vi "[FPGA] eHS Main (9039).vi"() -> ()   [LabVIEW 2017]
uses:
  <vilib>/OPAL-RT/eHS Toolkit/eHS Common/Controls/eHSx64 Gen3 Configuration.ctl
  <vilib>/OPAL-RT/Utilities Toolkit/Mapping/Input Mapping/FPGA/Controls/Input Mapping Configuration FIFO.ctl
  <vilib>/OPAL-RT/Utilities Toolkit/Mapping/Switch Mapping/FPGA/Controls/Switch Mapping Configuration FIFO.ctl
  <vilib>/OPAL-RT/Analog I-O Mapping & Conditioning Toolkit/AOMC/FPGA/Public/Controls/AOMC Configuration FIFO.ctl
  <vilib>/Platform/TimedLoop/XDataNode/timing_clust.ctl
  <vilib>/Platform/TimedLoop/XDataNode/nitl_modes.ctl
  <vilib>/Platform/TimedLoop/XDataNode/wakeup.ctl
  <vilib>/OPAL-RT/Analog I-O Mapping & Conditioning Toolkit/AIC/FPGA/Public/Controls/AIC Configuration FIFO.ctl
  <vilib>/OPAL-RT/FPGA Signal Generation Toolkit/Sinewave Generation/FPGA/Public/Controls/Sinewave Configuration FIFO.ctl
  <vilib>/OPAL-RT/FPGA Signal Generation Toolkit/SPWM Generation/FPGA/Public/Controls/SPWM Configuration FIFO.ctl
  <vilib>/OPAL-RT/FPGA Signal Generation Toolkit/PWM Generation/FPGA/Public/Controls/PWM Configuration FIFO.ctl
  <vilib>/OPAL-RT/Analog I-O Mapping & Conditioning Toolkit/AOMC/FPGA/Public/Controls/Input Sources.ctl
  <vilib>/OPAL-RT/Utilities Toolkit/Mapping/Input Mapping/FPGA/Controls/Sources/Input Sources - Parallelx32.ctl
  <vilib>/OPAL-RT/Utilities Toolkit/Mapping/Switch Mapping/FPGA/Controls/Sources/Switch Sources - Parallelx72.ctl
  <vilib>/rvi/Emulation/niFpgaGetClockAttributes.vi
  <vilib>/rvi/Emulation/niFpgaSctlEmulationGetInTimedLoop.vi
  <vilib>/rvi/Emulation/niFpgaEmulationReportErrorSimple.vi
  <vilib>/OPAL-RT/Utilities Toolkit/Mapping/Input Mapping/FPGA/SubVIs/Initialize/Initialize Input Mapping - Parallelx32.vi
  <vilib>/OPAL-RT/Utilities Toolkit/Mapping/Switch Mapping/FPGA/SubVIs/Initailize/Initialize Switch Mapping - Parallelx72.vi
  <vilib>/rvi/DataTransferAndStorage/Container/Common/niFpgaContainerExecOnDevCompGetState.vi
  <vilib>/rvi/Emulation/niFpgaEmulationIsFPGAContextNoSignature.vi
  <vilib>/rvi/DataTransferAndStorage/Container/Common/niFpgaContainerGetUniqueNameForEmu.vi
  <vilib>/rvi/Memory/Memory_Emulation/niFpgaMemoryEmulationCacheClearOnFirstRun.vi
  <vilib>/rvi/Memory/Memory_Emulation/nirvimemoryEmulationManagerCache_MakeExclusive.vi
  <vilib>/rvi/Memory/Memory_Emulation/niFpgaMemoryEmulationValidateCache.vi
  <vilib>/rvi/Memory/Memory_Emulation/nirvimemoryEmulationManagerCache_InsertValue.vi
  <vilib>/Utility/error.llb/Clear Errors.vi
  <vilib>/rvi/Memory/Memory_Emulation/nirvimemoryEmulationManagerCache_ReleaseExclusive.vi
  <vilib>/rvi/Memory/Memory_Emulation/nirvimemoryEmulationManagerCache_GetValue.vi
  <vilib>/rvi/Memory/Memory_Emulation/nirvimemoryEmulationManagerCache_SetValue.vi
  <vilib>/rvi/Emulation/niFpgaProcessEmulError.vi
  <vilib>/rvi/eio/common/nirviEmuTemplateMethod_errors.vi
  <vilib>/rvi/Emulation/niFpgaCriticalErrorInLSC.vi
  <vilib>/OPAL-RT/FPGA Signal Generation Toolkit/Sinewave Generation/FPGA/Private/Generators/Sinewave Generators (32-CH Parallel).vi
  <vilib>/OPAL-RT/FPGA Signal Generation Toolkit/SPWM Generation/FPGA/Private/Generators/SPWM Generators (12-CH Parallel).vi
  <vilib>/OPAL-RT/FPGA Signal Generation Toolkit/PWM Generation/FPGA/Private/Generators/PWM Generators (16-CH Parallel).vi
  <vilib>/OPAL-RT/Analog I-O Mapping & Conditioning Toolkit/AOMC/FPGA/Private/AO Mapping & Conditioning (FXP(20,5)).vi
  <vilib>/OPAL-RT/Analog I-O Mapping & Conditioning Toolkit/AIC/FPGA/Private/AI Conditioning FXP(20,5).vi
  <vilib>/OPAL-RT/eHS Toolkit/eHS FPGA/SubVIs/eHSx64 Gen3 Solver Core.vi
  <vilib>/OPAL-RT/Utilities Toolkit/Mapping/Switch Mapping/FPGA/SubVIs/Configure/Get Switch Mapping Configuration from Host - Parallelx72.vi
  <vilib>/OPAL-RT/Utilities Toolkit/Mapping/Input Mapping/FPGA/SubVIs/Configure/Get Input Mapping Configuration from Host - Parallelx32.vi
  <vilib>/OPAL-RT/Utilities Toolkit/Mapping/Switch Mapping/FPGA/SubVIs/Map/Map Switches - Parallelx72.vi
  <vilib>/OPAL-RT/Utilities Toolkit/Mapping/Input Mapping/FPGA/SubVIs/Map/Map Inputs - Parallelx32.vi
  <vilib>/rvi/interface/RandomDataEmulation/niFpgaRandomDataHandleErrors.vi
  <vilib>/Platform/TimedLoop/XDataNode/XDataNode.xnode
  <vilib>/rvi/DataTransferAndStorage/Container/XNode/niFpgaContainer.xnode
  <vilib>/rvi/DataTransferAndStorage/Register/Emulation/niFpgaRegisterEmulationRefIn.vi
  <vilib>/eio/EIONode/EIONode.xnode
  <vilib>/rvi/interface/RandomDataEmulation/nirviRandomDataFpgaReadWriteTemplate.vi
  <vilib>/Platform/TimedLoop/XDataNode/XDNodeRunTimeDep.lvlib
  <vilib>/OPAL-RT/Utilities Toolkit/Mapping/Input Mapping/FPGA/Input Mapping - FPGA.lvlib
  <vilib>/OPAL-RT/Utilities Toolkit/Mapping/Switch Mapping/FPGA/Switch Mapping - FPGA.lvlib
  <vilib>/OPAL-RT/Analog I-O Mapping & Conditioning Toolkit/AOMC/FPGA/AO Mapping & Conditioning - FPGA.lvlib
  <vilib>/OPAL-RT/Analog I-O Mapping & Conditioning Toolkit/AIC/FPGA/AI Conditioning - FPGA.lvlib
  <vilib>/OPAL-RT/eHS Toolkit/eHS FPGA/eHS - FPGA.lvlib
  <vilib>/OPAL-RT/Utilities Toolkit/Utilities/Type Casting/FPGA/Type Casting - FPGA.lvlib
  <vilib>/OPAL-RT/FPGA Signal Generation Toolkit/Sinewave Generation/FPGA/Sinewave Generation - FPGA.lvlib
  <vilib>/OPAL-RT/FPGA Signal Generation Toolkit/SPWM Generation/FPGA/SPWM Generation - FPGA.lvlib
  <vilib>/OPAL-RT/FPGA Signal Generation Toolkit/PWM Generation/FPGA/PWM Generation - FPGA.lvlib
  <vilib>/OPAL-RT/eHS Toolkit/eHS Common/eHS - Common.lvlib
panel:
  in  "View SPWM":bool
  in  "Mod Index":fxp<+/-,32,2>
  in  "Carrier Frequency":fxp<+/-,32,1>=0.00039999978616833687
  in  "Reset Sinewaves?":bool
  in  "Auto-Synchronize Sinewaves?":bool
  in  "Auto-Synchronize SPWM?":bool
  in  "Reset SPWMs?":bool
  in  "Reset PWMs?":bool
  out "Conditioned AI Data_Debug":sgl[](array[numeric])
  out "Mapped & Conditioned Data_Debug":fxp<+/-,20,5>[](array[numeric])
  in  "eHS Switches (CPU)":bool[](array[boolean])=[FALSE, FALSE, FALSE, FALSE, FALSE, FALSE, FALSE, FALSE, FALSE, FALSE, FALSE, FALSE, FALSE, FALSE, FALSE, FALSE, FALSE, FALSE, FALSE, FALSE, FALSE, FALSE, FALSE, FALSE, FALSE, FALSE, FALSE, FALSE, FALSE, FALSE, FALSE, FALSE, FALSE, FALSE, FALSE, FALSE, FALSE, FALSE, FALSE, FALSE, FALSE, FALSE, FALSE, FALSE, FALSE, FALSE, FALSE, FALSE, FALSE, FALSE, FALSE, FALSE, FALSE, FALSE, FALSE, FALSE, FALSE, FALSE, FALSE, FALSE, FALSE, FALSE, FALSE, FALSE, FALSE, FALSE, FALSE, FALSE, FALSE, FALSE, FALSE, FALSE]
  in  "eHS Input (CPU)":u32[](array[numeric])=[0, 0, 0, 0, 0, 0, 0, 0, 0, 0, 0, 0, 0, 0, 0, 0, 0, 0, 0, 0, 0, 0, 0, 0, 0, 0, 0, 0, 0, 0, 0, 0]
  in  "eHSx64 Gen3 Configuration":T1
  out "Finished":bool
  in  "stop":bool
  out "Module Underflow":bool
  out "Acq Loop Ticks":u32
  out "DMA FIFO Full":bool
  out "Chan Count":bool
  out "First Read":bool
  in  "Number of Channels":i32=4
  in  "Samps per Chan [Finite]":i32=5120
  in  "Acquisition Type":enum16{"Finite Samples", "Continuous Samples"}(ring)
  out "oclk div":u32
  out "oclk freq":u32
  in  "data rate (S/s)":u32
  out "oclk mult":u32
  out "FPGA Error":errorcluster
  in  "Chan Scale Array":sgl[](array[numeric])=[0.0, 0.0, 0.0, 0.0, 0.0, 0.0, 0.0, 0.0, 0.0, 0.0, 0.0, 0.0, 0.0, 0.0, 0.0, 0.0, 0.0, 0.0, 0.0, 0.0, 0.0, 0.0, 0.0, 0.0, 0.0, 0.0, 0.0, 0.0, 0.0, 0.0, 0.0, 0.0, 0.0, 0.0, 0.0, 0.0, 0.0, 0.0, 0.0, 0.0]
  # "Signal Generation Paramters"
  # "eHS Parameters"
  # "RIO Waveform Parameters"
  # "Debug"
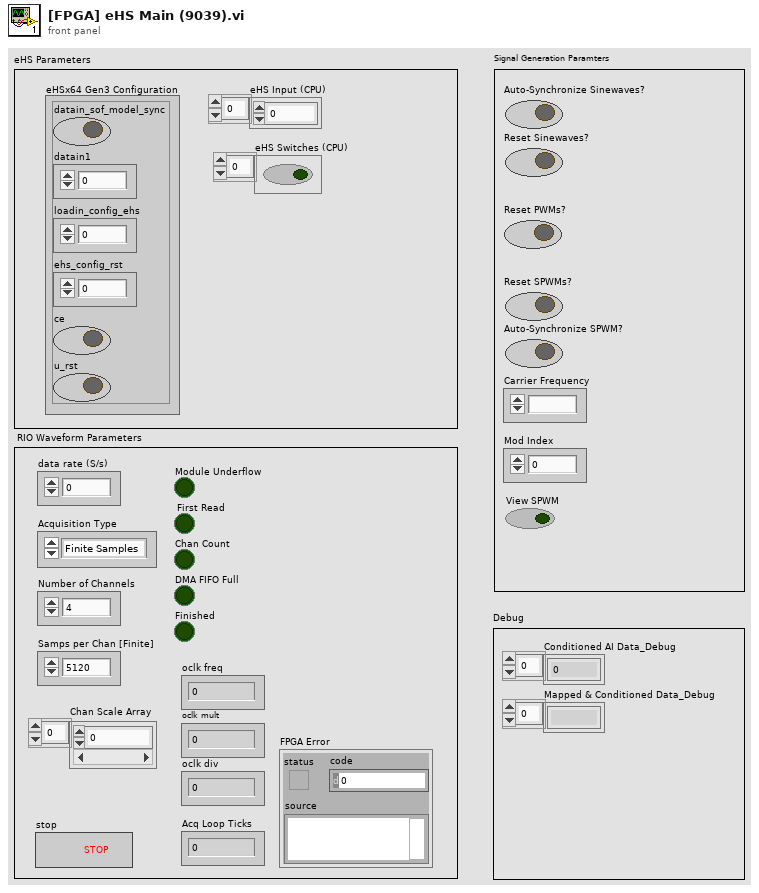
[diagram p1: front panel]
types:
  T1 = typedef "OPAL-RT eHS.lvlib/eHS - Common.lvlib/eHSx64 Gen3 Configuration.ctl" = cluster{"datain_sof_model_sync":bool, "datain1":fxp<+,33,33>, "loadin_config_ehs":fxp<+,33,33>, "ehs_config_rst":fxp<+,33,33>, "ce":bool, "u_rst":bool}
  T2 = typedef "PWM Generation - FPGA.lvlib/PWM Configuration FIFO.ctl" = refnum<k21>
  T3 = typedef "SPWM Generation - FPGA.lvlib/SPWM Configuration FIFO.ctl" = refnum<k21>
  T4 = typedef "Sinewave Generation - FPGA.lvlib/Sinewave Configuration FIFO.ctl" = refnum<k21>
  T5 = typedef "AI Conditioning - FPGA.lvlib/AIC Configuration FIFO.ctl" = refnum<k21>
  T6 = typedef "AO Mapping & Conditioning - FPGA.lvlib/AOMC Configuration FIFO.ctl" = refnum<k21>
  T7 = typedef "Switch Mapping - FPGA.lvlib/Switch Mapping Configuration FIFO.ctl" = refnum<k21>
  T8 = typedef "Input Mapping - FPGA.lvlib/Input Mapping Configuration FIFO.ctl" = refnum<k21>
  T9 = typedef "[FPGA] Local FPGA Memory.ctl" = cluster{"Analog Inputs":refnum<k21>, "Conditioned AI":refnum<k21>, "Analog Outputs (FXP(20,5))":refnum<k21>, "Analog Outputs (U16)":refnum<k21>, "Digital Inputs":refnum<k21>, "Digital Outputs":refnum<k21>, "eHS Outputs - Lane 1":refnum<k21>, "eHS Outputs - Lane 2":refnum<k21>, "eHS Outputs - Lane 3":refnum<k21>, "SWG Signals":refnum<k21>, "PWM Signals":refnum<k21>, "SPWM Signals":refnum<k21>}
  T10 = typedef "XDNodeRunTimeDep.lvlib/timing_clust.ctl" = cluster{"Expected End [f-1]":u64, "Actual End [f-1]":u64, "Finished Late? [f-1]":bool, "Expected End [i-1]":u64, "Actual End [i-1]":u64, "Finished Late? [i-1]":bool, "Expected Start [i]":u64, "Actual Start [i]":u64, "Expected Start [f]":u64, "Actual Start [f]":u64, "Source Name":string, "Structure Name":string, "Period":i64, "Deadline":i64, "Offset":i64, "Start":i64, "Priority":i32, "Timeout":i32, "Mode":T11, "Wakeup Reason":T12, "Error":errorcluster, "Source Type":string, "Secondary Source Type":string, "Global End Time":u64, "Global Start Time":u64, "Frame Duration":u64, "Iteration Duration":u64, "Assigned CPU":i32, "I/O Scan Engine Mode":u32}
  T11 = typedef "XDNodeRunTimeDep.lvlib/nitl_modes.ctl" = enum32{"No Change", "Process missed periods, maintain original phase", "Discard missed periods, maintain original phase", "Process missed periods, ignore original phase", "Discard missed periods, ignore original phase"}
  T12 = typedef "XDNodeRunTimeDep.lvlib/wakeup.ctl" = enum32{"Normal", "Aborted", "Asynchronous wakeup", "Timing source error", "Timed loop error", "Timeout"}
  T13 = typedef "Sinewave Generation - FPGA.lvlib/Sinewave Generator FPGA Resources.ctl" = cluster{"Sinewave Configuration FIFO":T4, "Sinewave Configuration Memory":T14}
  T14 = typedef "Sinewave Generation - FPGA.lvlib/Sinewave Generator Memory.ctl" = cluster{"Sinewave Generator Configuration Memory":cluster{"Sinewave Generator Configuration - Buffer 0":refnum<k21>, "Sinewave Generator Configuration - Buffer 1":refnum<k21>}, "Frequency Engine Rate Memory":T15, "Frequency Engine Values Memory":T16, "Sinewave LUT Memory":T17}
  T15 = typedef "Signal Generation Utilities - FPGA.lvlib/Frequency Engine Rate Memory.ctl" = cluster{"Frequency Engine Rates - Buffer 0":refnum<k21>, "Frequency Engine Rates - Buffer 1":refnum<k21>}
  T16 = typedef "Signal Generation Utilities - FPGA.lvlib/Frequency Engine Values Memory.ctl" = cluster{"Frequency Engine Values - Buffer 0":refnum<k21>, "Frequency Engine Values - Buffer 1":refnum<k21>}
  T17 = typedef "Signal Generation Utilities - FPGA.lvlib/Sinewave LUT Memory.ctl" = cluster{"Sinewave LUT (SGL)":refnum<k21>, "Sinewave LUT (16,1)":refnum<k21>}
  T18 = typedef "SPWM Generation - FPGA.lvlib/SPWM Generator FPGA Resources.ctl" = cluster{"SPWM Configuration FIFO":T3, "SPWM Generator Memory":T19}
  T19 = typedef "SPWM Generation - FPGA.lvlib/SPWM Generator Memory.ctl" = cluster{"SPWM Configuration Parameters Memory":T20, "Frequency Engine Rate Memory":T15, "Frequency Engine Values Memory":T16, "Sinewave LUT Memory":T17}
  T20 = typedef "SPWM Generation - FPGA.lvlib/SPWM Configuration Parameters Memory.ctl" = cluster{"SPWM Generator Configuration - Buffer 0":refnum<k21>, "SPWM Generator Configuration - Buffer 1":refnum<k21>}
  T21 = typedef "PWM Generation - FPGA.lvlib/PWM Generator FPGA Resources.ctl" = cluster{"PWM Generator Memory":T22, "PWM Configuration FIFO":T2}
  T22 = typedef "PWM Generation - FPGA.lvlib/PWM Generator Memory.ctl" = cluster{"PWM Generation Configuration":refnum<k21>, "PWM Generator States":refnum<k21>}
  T23 = typedef "Input Mapping - FPGA.lvlib/Input Mapping FPGA Resources.ctl" = cluster{"Input Mapping Configuration FIFO":T8, "Input Mapping Configuration Memory":T24}
  T24 = typedef "Input Mapping - FPGA.lvlib/Input Mapping Configuration Memory.ctl" = cluster{"Input Mapping Memory - Lane 0":refnum<k21>, "Input Mapping Memory - Lane 1":refnum<k21>, "Input Mapping Memory - Lane 2":refnum<k21>, "Input Mapping Memory - Lane 3":refnum<k21>}
  T25 = typedef "Switch Mapping - FPGA.lvlib/Switch Mapping FPGA Resources.ctl" = cluster{"Switch Mapping Configuration FIFO":T7, "Switch Mapping Configuration Memory":T26}
  T26 = typedef "Switch Mapping - FPGA.lvlib/Switch Mapping Configuration Memory.ctl" = cluster{"Switch Mapping Memory - Lane 0":refnum<k21>, "Switch Mapping Memory - Lane 1":refnum<k21>, "Switch Mapping Memory - Lane 2":refnum<k21>, "Switch Mapping Memory - Lane 3":refnum<k21>, "Switch Mapping Memory - Lane 4":refnum<k21>, "Switch Mapping Memory - Lane 5":refnum<k21>, "Switch Mapping Memory - Lane 6":refnum<k21>, "Switch Mapping Memory - Lane 7":refnum<k21>, "Switch Mapping Memory - Lane 8":refnum<k21>}
  T27 = typedef "AI Conditioning - FPGA.lvlib/AIC FPGA Resources.ctl" = cluster{"AIC Configuration FIFO":T5, "AIC Memory":T28}
  T28 = typedef "AI Conditioning - FPGA.lvlib/AIC Memory.ctl" = cluster{"AIC Configuration Parameters":refnum<k21>}
  T29 = typedef "AO Mapping & Conditioning - FPGA.lvlib/AOMC FPGA Resources.ctl" = cluster{"AOMC Memory":T30, "AOMC Configuration FIFO":T6}
  T30 = typedef "AO Mapping & Conditioning - FPGA.lvlib/AOMC Memory.ctl" = cluster{"AOMC Configuration Parameters":refnum<k21>}
  T31 = typedef "Sinewave Generation - FPGA.lvlib/Sinewave Generator Parameters.ctl" = cluster{"Number of Sinewaves to Generate":u8, "Read Buffer Index":u8, "Reset Sinewaves?":bool}
  T32 = typedef "SPWM Generation - FPGA.lvlib/SPWM FPGA Generator Parameters.ctl" = cluster{"Carrier Frequency":fxp<+/-,32,1>, "Mod Index ":fxp<+/-,32,2>, "Number of SPWMs to Generate":u8, "Reset SPWMs?":bool, "Read Buffer Index":u8}
  T33 = typedef "PWM Generation - FPGA.lvlib/PWM Generator Parameters.ctl" = cluster{"Number of PWMs to Generate":u8, "Reset PWMs?":bool}
  T34 = typedef "Switch Mapping - FPGA.lvlib/Switch Sources - Parallelx72.ctl" = cluster{"Group A":bool[], "Group B":bool[], "Group C":bool[], "Group D":bool[], "Group E":bool[]}
  T35 = typedef "Input Mapping - FPGA.lvlib/Input Sources - Parallelx32.ctl" = cluster{"Group A":u32[], "Group B":u32[], "Group C":u32[], "Group D":u32[]}
  T36 = typedef "AO Mapping & Conditioning - FPGA.lvlib/Input Sources.ctl" = cluster{"Group A":sgl[], "Group B":sgl[]}
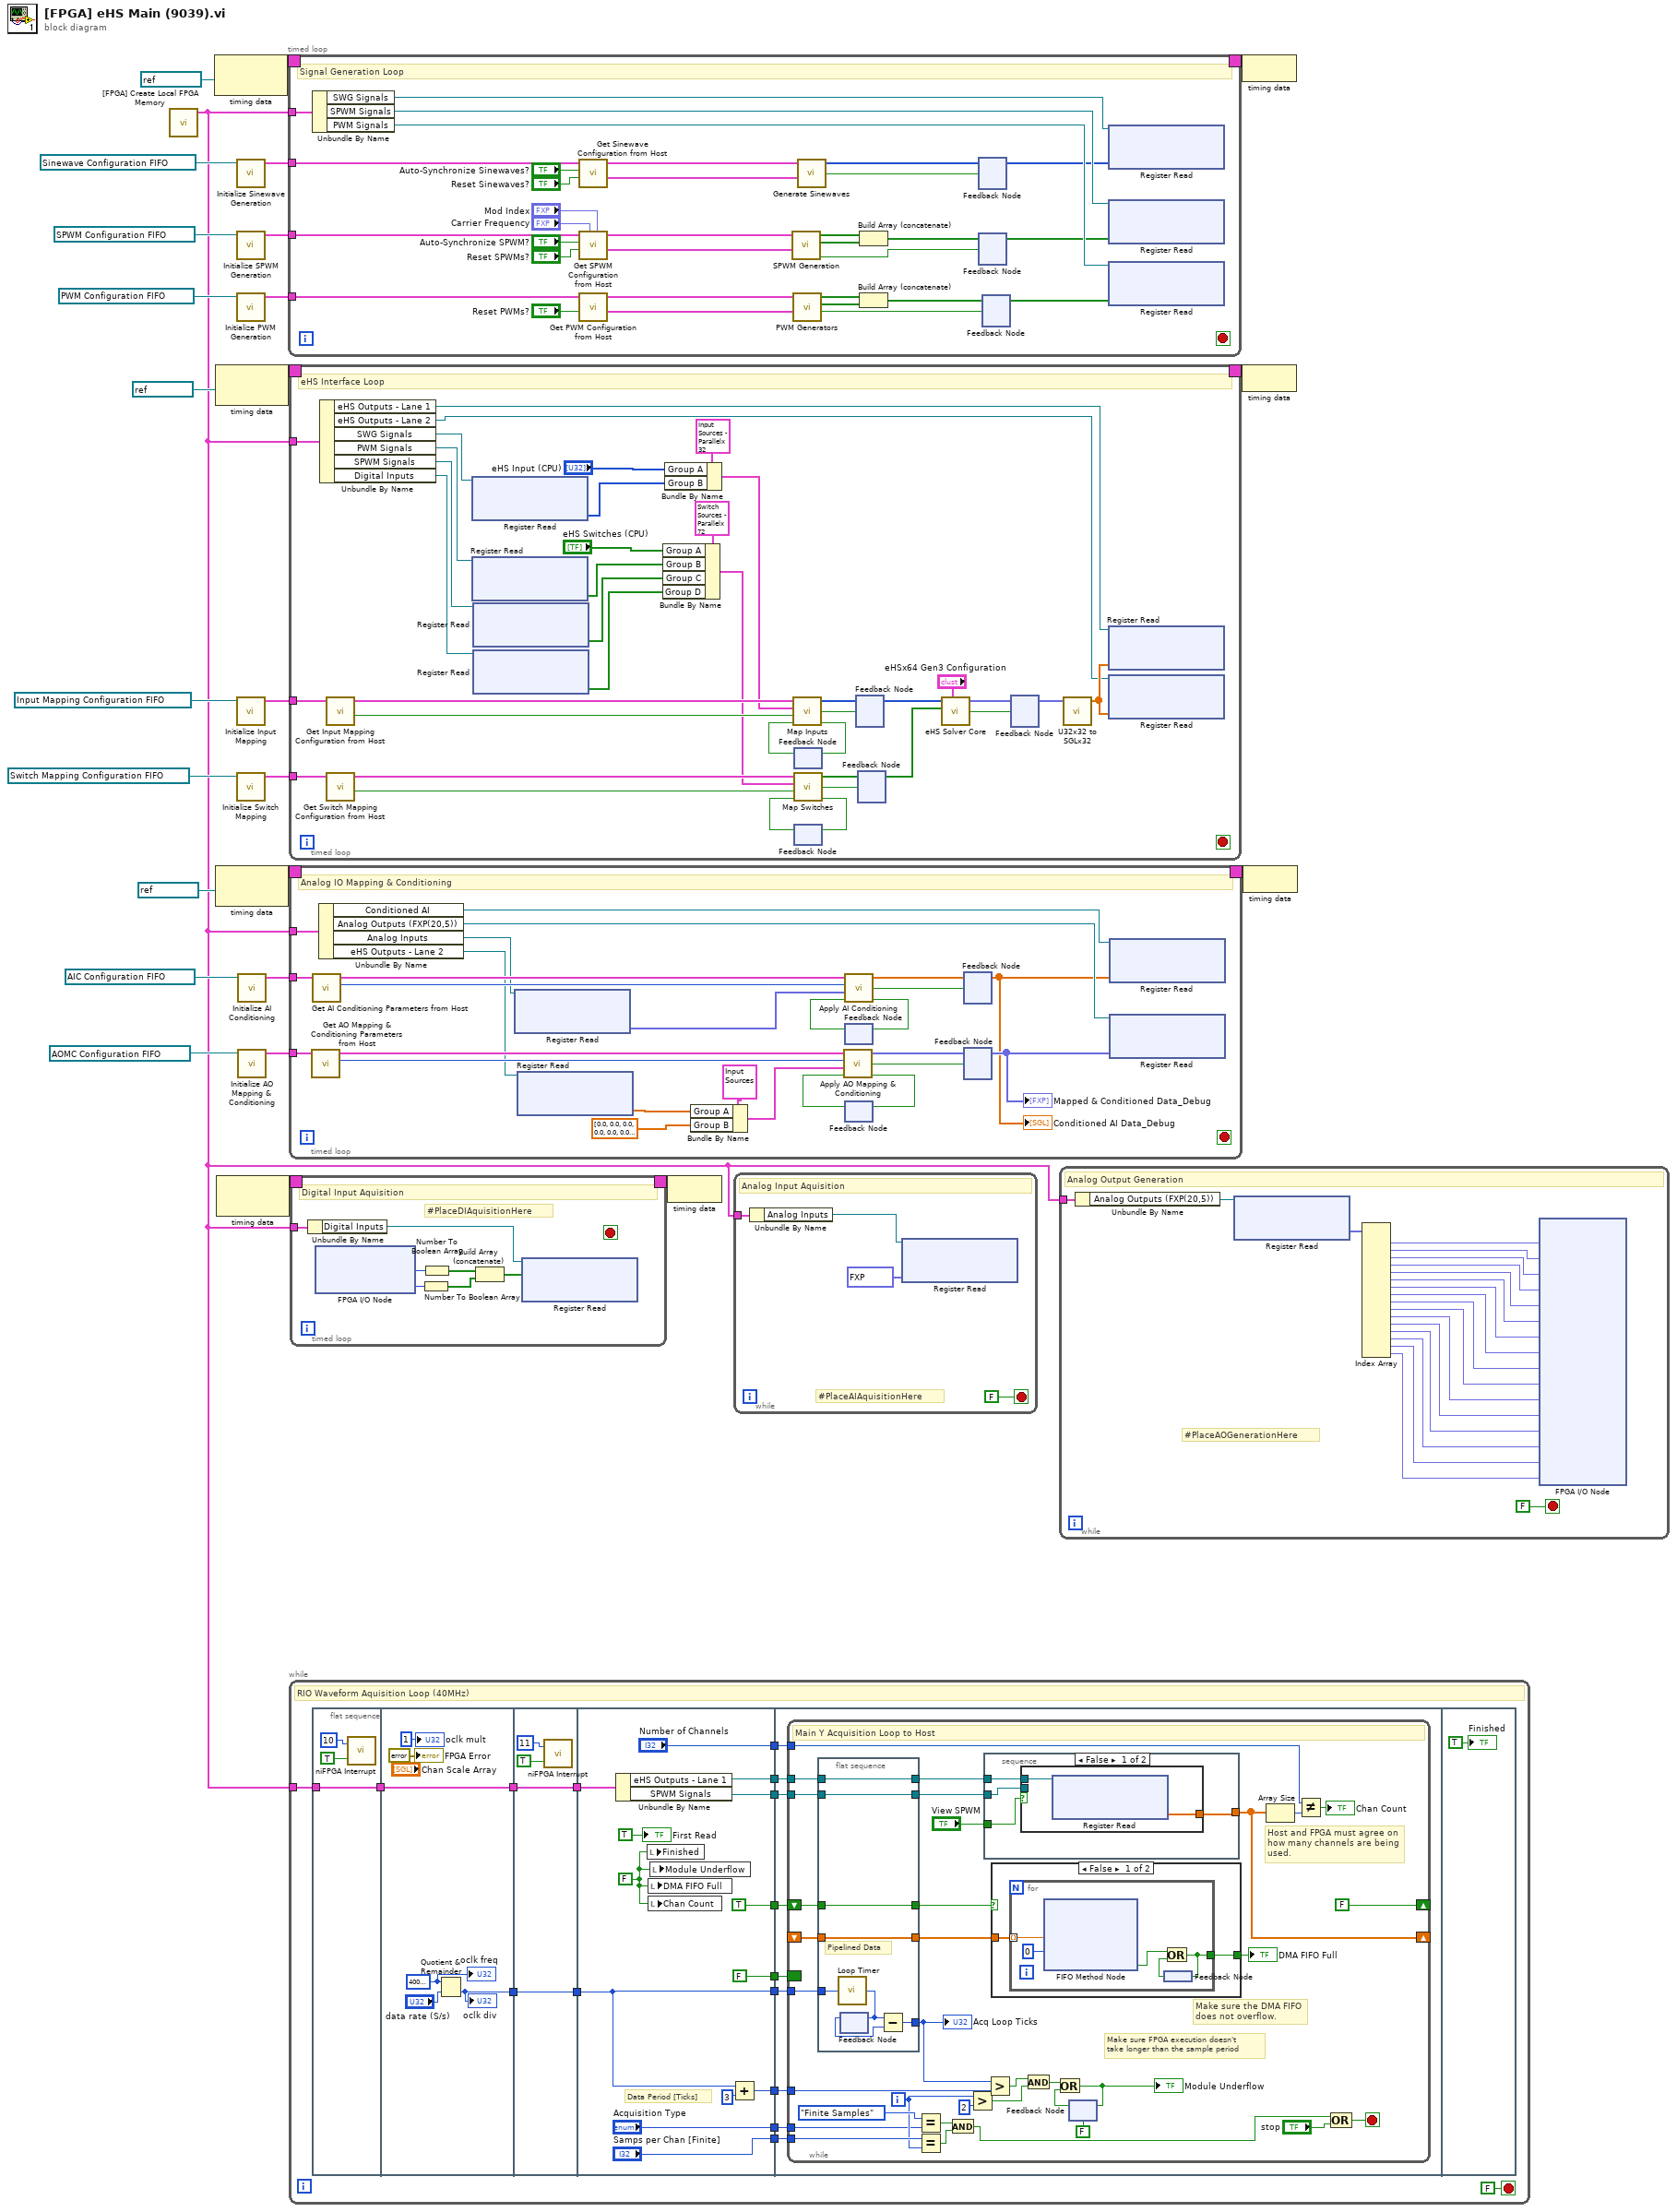
[diagram p0: block diagram]
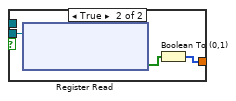
[diagram p2: hidden frame]
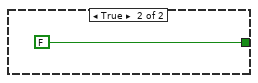
[diagram p3: hidden frame]
diagram:
  n1 = call "[FPGA] Create Local FPGA Memory.vi"() -> ("FPGA Memory"=w1:T9)  [unwired: 11 in]
  n2 = node-c288(refnum<k21> "100MHz" ("Source Name")) -> (w12:T10)
  n3 = node-c288(refnum<k21> "200MHz" ("Source Name")) -> (w26:T10)
  n4 = node-c288(refnum<k21> "200MHz" ("Source Name")) -> (w20:T10)
  n5 = node-c288() -> (w3:T10)  [unwired: 1 in]
  n6 = call <vilib>:"Initialize Sinewave Generation.vi"("Sinewave Configuration FIFO"=T4 "Sinewave Configuration FIFO") -> ("Sinewave Generator FPGA Resources"=w4:T13)  [unwired: 10 in]
  n7 = call <vilib>:"Initialize SPWM Generation.vi"("SPWM Configuration FIFO"=T3 "SPWM Configuration FIFO") -> ("SPWM Generator FPGA Resources"=w5:T18)  [unwired: 10 in]
  n8 = call <vilib>:"Initialize PWM Generation.vi"("PWM Configuration FIFO"=T2 "PWM Configuration FIFO") -> ("PWM Generator FPGA Resources"=w6:T21)  [unwired: 10 in]
  n9 = call-poly <vilib>:"Initialize Input Mapping.vi"("Input Mapping Configuration FIFO"=T8 "Input Mapping Configuration FIFO") -> ("Input Mapping FPGA Resources"=w14:T23)  [unwired: 10 in]
  n10 = call-poly <vilib>:"Initialize Switch Mapping.vi"("Switch Mapping Configuration FIFO"=T7 "Switch Mapping Configuration FIFO") -> ("Switch Mapping FPGA Resources"=w13:T25)  [unwired: 10 in]
  n11 = call <vilib>:"Initialize AI Conditioning.vi"("AIC Configuration FIFO"=T5 "AIC Configuration FIFO") -> ("AIC FPGA Resources"=w16:T27)  [unwired: 10 in]
  n12 = call <vilib>:"Initialize AO Mapping & Conditioning.vi"("AOMC Configuration FIFO"=T6 "AOMC Configuration FIFO") -> ("AOMC FPGA Resources"=w15:T29)  [unwired: 10 in]
  n13 = timed-loop {
    timing: w12 -> [_]
    timing-out: [_] -> w11
    tunnel: w1 -> [w59]
    tunnel: w6 -> [w58]
    tunnel: w5 -> [w57]
    tunnel: w4 -> [w56]
    stop <- _ stop-if-true
    # "Signal Generation Loop"
    n14 = Unbundle By Name(w59) -> ("SWG Signals"=w42:refnum<k21>, "SPWM Signals"=w41:refnum<k21>, "PWM Signals"=w40:refnum<k21>)
    n15 = call <vilib>:"Get Sinewave Configuration from Host.vi"("Reset Sinewaves?"="Reset Sinewaves?", "Auto-Synchronize Sinewaves?"="Auto-Synchronize Sinewaves?", "Sinewave Generator FPGA Resources"=w56) -> ("Sinewave Generator Parameters"=w49:T31, "Sinewave Configuration Memory"=w50:T14)  [unwired: 7 in]
    n16 = call <vilib>:"Get SPWM Configuration from Host.vi"("Mod Index"="Mod Index", "Carrier Frequency"="Carrier Frequency", "Reset SPWMs?"="Reset SPWMs?", "Auto-Synchronize SPWM?"="Auto-Synchronize SPWM?", "SPWM Generator FPGA Resources"=w57) -> ("SPWM Generator Parameters"=w47:T32, "SPWM Generator Memory"=w48:T19)  [unwired: 5 in]
    n17 = call <vilib>:"Get PWM Configuration from Host.vi"("Reset PWMs?"="Reset PWMs?", "PWM Generator FPGA Resources"=w58) -> ("PWM Generator Parameters"=w45:T33, "PWM Generator Memory"=w46:T22)  [unwired: 8 in]
    n18 = call-poly <vilib>:"SPWM Generation.vi"("SPWM Generator Parameters"=w47, "SPWM Generator Memory"=w48) -> ("Output Valid"=w30:bool, "!SPWM States"=w35:bool[], "SPWM States"=w36:bool[])  [unwired: 7 in]
    n19 = call-poly <vilib>:"PWM Generators.vi"("PWM Generator Parameters"=w45, "PWM Generator Memory"=w46) -> ("Output Valid?"=w28:bool, "!PWM States"=w31:bool[], "PWM States"=w32:bool[])  [unwired: 7 in]
    n20 = call-poly <vilib>:"Generate Sinewaves.vi"("Sinewave Generator Parameters"=w49, "Sinewave Generator Memory"=w50) -> ("Output Valid?"=w38:bool, "Sinewave (SGL-as-U32)"=w39:u32[])  [unwired: 8 in]
    n21 = Build Array (concatenate)(w36, w35) -> (w34:bool[])
    n22 = Build Array (concatenate)(w32, w31) -> (w29:bool[])
    n23 = feedback-in #1(w39, w38) -> ()
    n24 = feedback #1() -> (w37:u32[])  [unwired: 1 in]
    n25 = feedback #2() -> (w33:bool[])  [unwired: 1 in]
    n26 = feedback-in #2(w34, w30) -> ()
    n27 = feedback #3() -> (w27:bool[])  [unwired: 1 in]
    n28 = feedback-in #3(w29, w28) -> ()
    n29 = xnode ("Register Read")("Data"=w37, "Register In"=w42) -> ()  [unwired: 1 out]
    n30 = xnode ("Register Read")("Data"=w33, "Register In"=w41) -> ()  [unwired: 1 out]
    n31 = xnode ("Register Read")("Data"=w27, "Register In"=w40) -> ()  [unwired: 1 out]
  }
  n32 = timed-loop {
    timing: w26 -> [_]
    timing-out: [_] -> w25
    tunnel: w1 -> [w78]
    tunnel: w14 -> [w98]
    tunnel: w13 -> [w96]
    stop <- _ stop-if-true
    # "eHS Interface Loop"
    n33 = Unbundle By Name(w78) -> ("eHS Outputs - Lane 1"=w73:refnum<k21>, "eHS Outputs - Lane 2"=w70:refnum<k21>, "SWG Signals"=w69:refnum<k21>, "PWM Signals"=w68:refnum<k21>, "SPWM Signals"=w67:refnum<k21>, "Digital Inputs"=w63:refnum<k21>)
    n34 = call-poly <vilib>:"Get Input Mapping Configuration from Host.vi"("Input Mapping FPGA Resources"=w98) -> ("Settings Updated?"=w89:bool, "Input Mapping Configuration Memory"=w97:T24)  [unwired: 9 in]
    n35 = call-poly <vilib>:"Get Switch Mapping Configuration from Host.vi"("Switch Mapping FPGA Resources"=w96) -> ("Settings Updated?"=w90:bool, "Switch Mapping Configuration Memory"=w91:T26)  [unwired: 9 in]
    n36 = xnode ("Register Read")("Register In"=w69) -> ("Data"=w66:u32[])  [unwired: 1 out]
    n37 = xnode ("Register Read")("Register In"=w68) -> ("Data"=w65:bool[])  [unwired: 1 out]
    n38 = xnode ("Register Read")("Register In"=w67) -> ("Data"=w64:bool[])  [unwired: 1 out]
    n39 = xnode ("Register Read")("Register In"=w63) -> ("Data"=w62:bool[])  [unwired: 1 out]
    n40 = Bundle By Name(cluster=T34 {"Group A"=[FALSE, FALSE, FALSE, FALSE, FALSE, FALSE, FALSE, FALSE, FALSE, FALSE, FALSE, FALSE, FALSE, FALSE, FALSE, FALSE, FALSE, FALSE, FALSE, FALSE, FALSE, FALSE, FALSE, FALSE, FALSE, FALSE, FALSE, FALSE, FALSE, FALSE, FALSE, FALSE, FALSE, FALSE, FALSE, FALSE, FALSE, FALSE, FALSE, FALSE, FALSE, FALSE, FALSE, FALSE, FALSE, FALSE, FALSE, FALSE, FALSE, FALSE, FALSE, FALSE, FALSE, FALSE, FALSE, FALSE, FALSE, FALSE, FALSE, FALSE, FALSE, FALSE, FALSE, FALSE, FALSE, FALSE, FALSE, FALSE, FALSE, FALSE, FALSE, FALSE], "Group B"=[FALSE, FALSE, FALSE, FALSE, FALSE, FALSE, FALSE, FALSE, FALSE, FALSE, FALSE, FALSE, FALSE, FALSE, FALSE, FALSE, FALSE, FALSE, FALSE, FALSE, FALSE, FALSE, FALSE, FALSE, FALSE, FALSE, FALSE, FALSE, FALSE, FALSE, FALSE, FALSE, FALSE, FALSE, FALSE, FALSE, FALSE, FALSE, FALSE, FALSE, FALSE, FALSE, FALSE, FALSE, FALSE, FALSE, FALSE, FALSE, FALSE, FALSE, FALSE, FALSE, FALSE, FALSE, FALSE, FALSE, FALSE, FALSE, FALSE, FALSE, FALSE, FALSE, FALSE, FALSE, FALSE, FALSE, FALSE, FALSE, FALSE, FALSE, FALSE, FALSE], "Group C"=[FALSE, FALSE, FALSE, FALSE, FALSE, FALSE, FALSE, FALSE, FALSE, FALSE, FALSE, FALSE, FALSE, FALSE, FALSE, FALSE, FALSE, FALSE, FALSE, FALSE, FALSE, FALSE, FALSE, FALSE, FALSE, FALSE, FALSE, FALSE, FALSE, FALSE, FALSE, FALSE, FALSE, FALSE, FALSE, FALSE, FALSE, FALSE, FALSE, FALSE, FALSE, FALSE, FALSE, FALSE, FALSE, FALSE, FALSE, FALSE, FALSE, FALSE, FALSE, FALSE, FALSE, FALSE, FALSE, FALSE, FALSE, FALSE, FALSE, FALSE, FALSE, FALSE, FALSE, FALSE, FALSE, FALSE, FALSE, FALSE, FALSE, FALSE, FALSE, FALSE], "Group D"=[FALSE, FALSE, FALSE, FALSE, FALSE, FALSE, FALSE, FALSE, FALSE, FALSE, FALSE, FALSE, FALSE, FALSE, FALSE, FALSE, FALSE, FALSE, FALSE, FALSE, FALSE, FALSE, FALSE, FALSE, FALSE, FALSE, FALSE, FALSE, FALSE, FALSE, FALSE, FALSE, FALSE, FALSE, FALSE, FALSE, FALSE, FALSE, FALSE, FALSE, FALSE, FALSE, FALSE, FALSE, FALSE, FALSE, FALSE, FALSE, FALSE, FALSE, FALSE, FALSE, FALSE, FALSE, FALSE, FALSE, FALSE, FALSE, FALSE, FALSE, FALSE, FALSE, FALSE, FALSE, FALSE, FALSE, FALSE, FALSE, FALSE, FALSE, FALSE, FALSE], "Group E"=[FALSE, FALSE, FALSE, FALSE, FALSE, FALSE, FALSE, FALSE, FALSE, FALSE, FALSE, FALSE, FALSE, FALSE, FALSE, FALSE, FALSE, FALSE, FALSE, FALSE, FALSE, FALSE, FALSE, FALSE, FALSE, FALSE, FALSE, FALSE, FALSE, FALSE, FALSE, FALSE, FALSE, FALSE, FALSE, FALSE, FALSE, FALSE, FALSE, FALSE, FALSE, FALSE, FALSE, FALSE, FALSE, FALSE, FALSE, FALSE, FALSE, FALSE, FALSE, FALSE, FALSE, FALSE, FALSE, FALSE, FALSE, FALSE, FALSE, FALSE, FALSE, FALSE, FALSE, FALSE, FALSE, FALSE, FALSE, FALSE, FALSE, FALSE, FALSE, FALSE]} ("Switch Sources"), "Group A"="eHS Switches (CPU)", "Group B"=w65, "Group C"=w64, "Group D"=w62) -> (w86:T34)
    n41 = Bundle By Name(cluster=T35 {"Group A"=[0, 0, 0, 0, 0, 0, 0, 0, 0, 0, 0, 0, 0, 0, 0, 0, 0, 0, 0, 0, 0, 0, 0, 0, 0, 0, 0, 0, 0, 0, 0, 0], "Group B"=[0, 0, 0, 0, 0, 0, 0, 0, 0, 0, 0, 0, 0, 0, 0, 0, 0, 0, 0, 0, 0, 0, 0, 0, 0, 0, 0, 0, 0, 0, 0, 0], "Group C"=[0, 0, 0, 0, 0, 0, 0, 0, 0, 0, 0, 0, 0, 0, 0, 0, 0, 0, 0, 0, 0, 0, 0, 0, 0, 0, 0, 0, 0, 0, 0, 0], "Group D"=[0, 0, 0, 0, 0, 0, 0, 0, 0, 0, 0, 0, 0, 0, 0, 0, 0, 0, 0, 0, 0, 0, 0, 0, 0, 0, 0, 0, 0, 0, 0, 0]} ("Input Sources"), "Group A"="eHS Input (CPU)", "Group B"=w66) -> (w85:T35)
    n42 = feedback #4() -> (w94:bool)  [unwired: 1 in]
    n43 = call-poly <vilib>:"Map Inputs.vi"("Input Valid?"=w94, "Settings Updated?"=w89, "Input Sources"=w85, "Input Mapping Configuration Memory"=w97) -> ("Ready for Input?"=w95:bool, "Output Valid?"=w84:bool, "Mapped Inputs"=w83:u32[])  [unwired: 5 in]
    n44 = feedback-in #4(w95) -> ()
    n45 = feedback #5() -> (w92:bool)  [unwired: 1 in]
    n46 = call-poly <vilib>:"Map Switches.vi"("Input Valid?"=w92, "Settings Updated?"=w90, "Switch Sources"=w86, "Switch Mapping Configuration Memory"=w91) -> ("Ready for Input?"=w93:bool, "Output Valid?"=w82:bool, "Mapped Switches"=w81:bool[])  [unwired: 5 in]
    n47 = feedback-in #5(w93) -> ()
    n48 = feedback #6() -> (w79:u32[])  [unwired: 1 in]
    n49 = feedback-in #6(w83, w84) -> ()
    n50 = feedback #7() -> (w80:bool[])  [unwired: 1 in]
    n51 = feedback-in #7(w81, w82) -> ()
    n52 = call-poly <vilib>:"eHS Solver Core.vi"("eHSx64 Gen3 Configuration"="eHSx64 Gen3 Configuration", "eHSx64 Switches (SW)"=w80, "eHSx64 Inputs (U)"=w79) -> ("Output Valid?"=w75:bool, "eHSx64 Outputs (Y)"=w74:fxp<+,32,32>[])  [unwired: 5 in, 2 out]
    n53 = feedback #8() -> (w72:fxp<+,32,32>[])  [unwired: 1 in]
    n54 = feedback-in #8(w74, w75) -> ()
    n55 = call <vilib>:"U32x32 to SGLx32.vi"("U32x32"=w72) -> ("SGLx32"=w71:sgl[])  [unwired: 10 in]
    n56 = xnode ("Register Read")("Data"=w71, "Register In"=w73) -> ()  [unwired: 1 out]
    n57 = xnode ("Register Read")("Data"=w71, "Register In"=w70) -> ()  [unwired: 1 out]
  }
  n58 = timed-loop {
    timing: w20 -> [_]
    timing-out: [_] -> w19
    tunnel: w1 -> [w121]
    tunnel: w16 -> [w125]
    tunnel: w15 -> [w124]
    stop <- _ stop-if-true
    # "Analog IO Mapping & Conditioning"
    n59 = call <vilib>:"Get AO Mapping & Conditioning Parameters from Host.vi"("AOMC FPGA Resources"=w124) -> ("Number of Active AO Channels"=w122:u8, "AOMC Memory"=w123:T30)  [unwired: 9 in]
    n60 = call <vilib>:"Get AI Conditioning Parameters from Host.vi"("AIC FPGA Resources"=w125) -> ("Number of Active AI Channels"=w127:u8, "AIC Memory"=w126:T28)  [unwired: 9 in]
    n61 = Unbundle By Name(w121) -> ("Conditioned AI"=w111:refnum<k21>, "Analog Outputs (FXP(20,5))"=w110:refnum<k21>, "Analog Inputs"=w113:refnum<k21>, "eHS Outputs - Lane 2"=w120:refnum<k21>)
    n62 = xnode ("Register Read")("Register In"=w113) -> ("Data"=w112:fxp<+/-,20,5>[])  [unwired: 1 out]
    n63 = xnode ("Register Read")("Register In"=w120) -> ("Data"=w104:sgl[])  [unwired: 1 out]
    n64 = Bundle By Name(cluster=T36 {"Group A"=[0.0, 0.0, 0.0, 0.0, 0.0, 0.0, 0.0, 0.0, 0.0, 0.0, 0.0, 0.0, 0.0, 0.0, 0.0, 0.0, 0.0, 0.0, 0.0, 0.0, 0.0, 0.0, 0.0, 0.0, 0.0, 0.0, 0.0, 0.0, 0.0, 0.0, 0.0, 0.0], "Group B"=[0.0, 0.0, 0.0, 0.0, 0.0, 0.0, 0.0, 0.0, 0.0, 0.0, 0.0, 0.0, 0.0, 0.0, 0.0, 0.0, 0.0, 0.0, 0.0, 0.0, 0.0, 0.0, 0.0, 0.0, 0.0, 0.0, 0.0, 0.0, 0.0, 0.0, 0.0, 0.0]} ("Solver Data"), "Group A"=w104, "Group B"=sgl[] [0.0, 0.0, 0.0, 0.0, 0.0, 0.0, 0.0, 0.0, 0.0, 0.0, 0.0, 0.0, 0.0, 0.0, 0.0, 0.0, 0.0, 0.0, 0.0, 0.0, 0.0, 0.0, 0.0, 0.0, 0.0, 0.0, 0.0, 0.0, 0.0, 0.0, 0.0, 0.0]) -> (w114:T36)
    n65 = feedback #9() -> (w118:bool)  [unwired: 1 in]
    n66 = call-poly <vilib>:"Apply AI Conditioning.vi"("Input Valid?"=w118, "AI Data"=w112, "Number of Supported AI Channels"=w127, "AIC Memory"=w126) -> ("Ready for Input?"=w119:bool, "Output Valid?"=w109:bool, "Conditioned AI Data"=w108:sgl[])  [unwired: 5 in]
    n67 = feedback-in #9(w119) -> ()
    n68 = feedback #10() -> (w116:bool)  [unwired: 1 in]
    n69 = call-poly <vilib>:"Apply AO Mapping & Conditioning.vi"("Input Valid?"=w116, "Data"=w114, "Number of Active AO Channels"=w122, "AOMC Memory"=w123) -> ("Ready for Input?"=w117:bool, "Output Valid?"=w106:bool, "Mapped & Conditioned Data"=w107:fxp<+/-,20,5>[])  [unwired: 5 in]
    n70 = feedback-in #10(w117) -> ()
    n71 = feedback #11() -> (w102:sgl[])  [unwired: 1 in]
    "Conditioned AI Data_Debug" <- w102
    n72 = feedback-in #11(w108, w109) -> ()
    n73 = feedback #12() -> (w105:fxp<+/-,20,5>[])  [unwired: 1 in]
    "Mapped & Conditioned Data_Debug" <- w105
    n74 = feedback-in #12(w107, w106) -> ()
    n75 = xnode ("Register Read")("Data"=w102, "Register In"=w111) -> ()  [unwired: 1 out]
    n76 = xnode ("Register Read")("Data"=w105, "Register In"=w110) -> ()  [unwired: 1 out]
  }
  n77 = while {
    tunnel: w1 -> [w134]
    stop <- FALSE stop-if-true
    # "RIO Waveform Aquisition Loop (40MHz)"
    n78 = flat-sequence {
      tunnel: w134 -> [w146]
      tunnel: [w146] -> w133
      tunnel: [w152] -> w139
      tunnel: w133 -> [w151]
      tunnel: [w151] -> w132
      tunnel: [w156] -> w140
      tunnel: w139 -> [w156]
      tunnel: [w155] -> w135
      tunnel: w132 -> [w155]
      tunnel: ["Number of Channels"] -> w145
      tunnel: ["Samps per Chan [Finite]"] -> w144
      tunnel: [w165] -> w143
      tunnel: [w166] -> w142
      tunnel: [TRUE] -> w141
      tunnel: w140 -> [w165]
      tunnel: [FALSE] -> w138
      tunnel: ["Acquisition Type"] -> w136
      tunnel: w135 -> [w161]
      tunnel: [w160] -> w131
      tunnel: [w159] -> w130
      tunnel: w145 -> [w180]
      tunnel: w144 -> [w178]
      tunnel: w143 -> [w179]
      tunnel: w142 -> [w177]
      tunnel: w141 -> [w176]
      tunnel: w138 -> [w175]
      tunnel: w136 -> [w174]
      tunnel: w131 -> [w173]
      tunnel: w130 -> [w172]
      frame #0 {
        n79 = call <vilib>:"niFPGA Interrupt.vi"("Wait Until Cleared (F)"=TRUE ("Wait Until Cleared"), "IRQ Number (0)"=u8 10 ("IRQ Number")) -> ()  [unwired: 1 in]
      }
      frame #1 {
        w153 = u32 40000000 ("oclk freq")
        n80 = Quotient & Remainder(x=w153, y="data rate (S/s)") -> (floor(x/y)=w152:u32)  [unwired: 1 out]
        "oclk div" <- w152
        "oclk freq" <- w153
        "oclk mult" <- u32 1 ("oclk mult")
        "FPGA Error" <- errorcluster {"status"=FALSE, "code"=0, "source"=""} ("FPGA Error")
      }
      frame #2 {
        n81 = call <vilib>:"niFPGA Interrupt.vi"("Wait Until Cleared (F)"=TRUE ("Wait Until Cleared"), "IRQ Number (0)"=u8 11 ("IRQ Number")) -> ()  [unwired: 1 in]
      }
      frame #3 {
        w170 = FALSE ("Module Underflow")
        # "Data Period [Ticks]"
        n82 = Unbundle By Name(w161) -> ("eHS Outputs - Lane 1"=w160:refnum<k21>, "SPWM Signals"=w159:refnum<k21>)
        n83 = local write "Finished"(w170) -> ()
        n84 = local write "DMA FIFO Full"(w170) -> ()
        n85 = local write "Chan Count"(w170) -> ()
        n86 = local write "Module Underflow"(w170) -> ()
        n87 = Add(x=w165, y=u32 3) -> (x+y=w166:u32)
        "First Read" <- TRUE ("First Read")
      }
      frame #4 {
        n88 = while {
          tunnel: w178 -> [w209]
          shift-right: [w194] -> _
          shift-left: _ -> [w204]
          tunnel: w180 -> [w187]
          tunnel: w179 -> [w208]
          tunnel: w177 -> [w206]
          shift-right: [FALSE] -> _
          shift-left: w176 -> [w190]
          border: w175 -> [_]
          tunnel: w174 -> [w192]
          tunnel: w173 -> [w188]
          tunnel: w172 -> [w182]
          i -> [w202]
          stop <- w212 stop-if-true
          # "Host and FPGA must agree on \nhow many channels are being\nused."
          # "Make sure the DMA FIFO\ndoes not overflow."
          # "Make sure FPGA execution doesn't\ntake longer than the sample period"
          # "Main Y Acquisition Loop to Host"
          n89 = flat-sequence {
            tunnel: w208 -> [w239]
            tunnel: [w236] -> w205
            tunnel: [w235] -> w193
            tunnel: w204 -> [w235]
            tunnel: [w234] -> w191
            tunnel: w190 -> [w234]
            tunnel: [w233] -> w189
            tunnel: w188 -> [w233]
            tunnel: [w232] -> w183
            tunnel: w182 -> [w232]
            frame #0 {
              # "Pipelined Data"
              n90 = call "Loop Timer"("Count(Ticks)"=w239) -> ("Tick Count(Ticks)"=w237:u32)
              n91 = feedback-in #13(w237) -> ()
              n92 = feedback #13() -> (w238:u32)  [unwired: 1 out]
              n93 = Subtract(x=w237, y=w238) -> (x-y=w236:u32)
            }
          }
          n94 = Equal?(x=enum16{"Finite Samples", "Continuous Samples"}."Finite Samples" ("y"), y=w192) -> (x = y?=w197:bool)
          n95 = Equal?(x=w209, y=w202) -> (x = y?=w196:bool)
          n96 = And(x=w197, y=w196) -> (x .and. y?=w195:bool)
          n97 = Greater?(x=w202, y=2) -> (0:w184:bool)
          n98 = stacked-sequence {
            tunnel: [w217] -> w194
            tunnel: w189 -> [w218]
            tunnel: w183 -> [w215]
            tunnel: "View SPWM" -> [w216]
            frame #0 {
              n99 = case shown="False" w216 {
                tunnel: w218 -> [w220 _]
                tunnel: [w219 w221] -> w217
                tunnel: w215 -> [_ w223]
                frame False {
                  n100 = xnode ("Register Read")("Register In"=w220) -> ("Data"=w219:sgl[])  [unwired: 1 out]
                }
                frame True {
                  n101 = xnode ("Register Read")("Register In"=w223) -> ("Data"=w222:bool[])  [unwired: 1 out]
                  n102 = Boolean To (0,1)(Boolean=w222) -> (0, 1=w221:i16[])
                }
              }
            }
          }
          n103 = Greater?(x=w205, y=w206) -> (0:w185:bool)
          n104 = case shown="False" w191 {
            tunnel: [w225 FALSE] -> w211
            tunnel: w193 -> [w224 _]
            frame False {
              n105 = for {
                tunnel: [w229] -> w225
                tunnel: w224 -> [w226] mode=indexing
                n106 = xnode ("FIFO Method Node")("Element"=w226, "Timeout"=0) -> ("Timed Out?"=w227:bool)  [unwired: 1 in, 1 out]
                n107 = feedback #14() -> (w230:bool)
                n108 = Or(x=w227, y=w230) -> (x .or. y?=w229:bool)
                n109 = feedback-in #14(w229) -> ()
              }
            }
            frame True {
            }
          }
          "DMA FIFO Full" <- w211
          n110 = And(x=w185, y=w184) -> (x .and. y?=w199:bool)
          n111 = feedback #15(FALSE) -> (w201:bool)
          n112 = Or(x=w199, y=w201) -> (x .or. y?=w198:bool)
          "Module Underflow" <- w198
          n113 = feedback-in #15(w198) -> ()
          n114 = Array Size(array=w194) -> (size(s)=w186:i32)
          n115 = Not Equal?(x=w187, y=w186) -> (x != y?=→"Chan Count":bool)
          n116 = Compound Arithmetic op=OR(w195, "stop") -> (w212:bool)
          "Acq Loop Ticks" <- w205
        }
      }
      frame #5 {
        "Finished" <- TRUE ("Finished")
      }
    }
  }
  n117 = timed-loop {
    timing: w3 -> [_]
    timing-out: [_] -> w2
    tunnel: w1 -> [w247]
    stop <- _ stop-if-true
    # "#PlaceDIAquisitionHere"
    # "Digital Input Aquisition"
    n118 = Unbundle By Name(w247) -> ("Digital Inputs"=w246:refnum<k21>)
    n119 = xnode "FPGA I/O Node"() -> ("Mod3/DIO7:0"=w244:u8, "Mod4/DIO7:0"=w243:u8)  [unwired: 2 in, 2 out]
    n120 = Number To Boolean Array(number=w243) -> (Boolean array=w241:bool[])
    n121 = Number To Boolean Array(number=w244) -> (Boolean array=w242:bool[])
    n122 = Build Array (concatenate)(w242, w241) -> (w245:bool[])
    n123 = xnode ("Register Read")("Data"=w245, "Register In"=w246) -> ()  [unwired: 1 out]
  }
  n124 = node-c288(w2) -> ()
  n125 = while {
    tunnel: w1 -> [w252]
    stop <- FALSE stop-if-true
    # "#PlaceAIAquisitionHere"
    # "Analog Input Aquisition"
    n126 = Unbundle By Name(w252) -> ("Analog Inputs"=w251:refnum<k21>)
    n127 = xnode ("Register Read")("Data"=fxp<+/-,20,5>[] [0.0, 0.0, 0.0, 0.0, 0.0, 0.0, 0.0, 0.0, 0.0, 0.0, 0.0, 0.0, 0.0, 0.0, 0.0, 0.0, 0.0, 0.0, 0.0, 0.0, 0.0, 0.0, 0.0, 0.0, 0.0, 0.0, 0.0, 0.0, 0.0, 0.0, 0.0, 0.0], "Register In"=w251) -> ()  [unwired: 1 out]
  }
  n128 = while {
    tunnel: w1 -> [w272]
    stop <- FALSE stop-if-true
    # "#PlaceAOGenerationHere"
    # "Analog Output Generation"
    n129 = Unbundle By Name(w272) -> ("Analog Outputs (FXP(20,5))"=w271:refnum<k21>)
    n130 = xnode ("Register Read")("Register In"=w271) -> ("Data"=w270:fxp<+/-,20,5>[])  [unwired: 1 out]
    n131 = Index Array(array=w270) -> (element #1=w269:fxp<+/-,20,5>, element #2=w268:fxp<+/-,20,5>, element #3=w267:fxp<+/-,20,5>, element #4=w266:fxp<+/-,20,5>, element #5=w265:fxp<+/-,20,5>, element #6=w264:fxp<+/-,20,5>, element #7=w263:fxp<+/-,20,5>, element #8=w262:fxp<+/-,20,5>, element #9=w261:fxp<+/-,20,5>, element #10=w260:fxp<+/-,20,5>, element #11=w259:fxp<+/-,20,5>, element #12=w258:fxp<+/-,20,5>, element #13=w257:fxp<+/-,20,5>, element #14=w256:fxp<+/-,20,5>, element #15=w255:fxp<+/-,20,5>, element #16=w254:fxp<+/-,20,5>)  [unwired: 16 in]
    n132 = xnode "FPGA I/O Node"("Mod2/AO0"=w269, "Mod2/AO1"=w268, "Mod2/AO2"=w267, "Mod2/AO3"=w266, "Mod5/AO0"=w265, "Mod5/AO1"=w264, "Mod5/AO2"=w263, "Mod5/AO3"=w262, "Mod6/AO0"=w261, "Mod6/AO1"=w260, "Mod6/AO2"=w259, "Mod6/AO3"=w258, "Mod7/AO0"=w257, "Mod7/AO1"=w256, "Mod7/AO2"=w255, "Mod7/AO3"=w254) -> ()  [unwired: 16 in, 16 out]
  }
  n133 = node-c288(w11) -> ()
  n134 = node-c288(w25) -> ()
  n135 = node-c288(w19) -> ()
